vi "Scale Output ADXL345.vi"(9 "Byte1":u8, 11 "Byte0":u8) -> (3 "G's":fxp<+/-,32,10>)   [LabVIEW 2015]
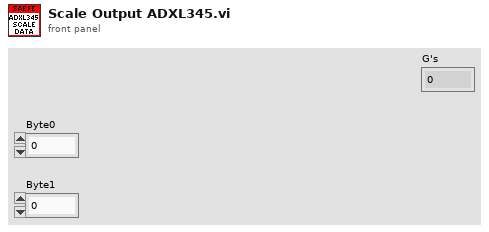
[diagram p1: front panel]
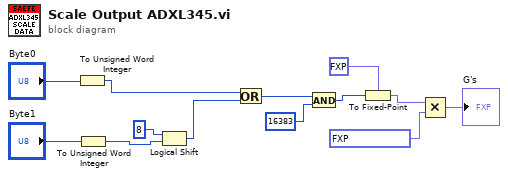
[diagram p0: block diagram]
diagram:
  n1 = To Unsigned Word Integer(number="Byte0") -> (unsigned 16bit integer=w9:u16)
  n2 = To Unsigned Word Integer(number="Byte1") -> (unsigned 16bit integer=w11:u16)
  n3 = Logical Shift(y=i16 8, x=w11) -> (x << y=w8:u16)
  n4 = Or(x=w9, y=w8) -> (x .or. y?=w7:u16)
  n5 = And(x=w7, y=u16 16383) -> (x .and. y?=w3:u16)
  n6 = To Fixed-Point(fixed-point type=fxp<+/-,16,16> 0.0, number=w3) -> (fixed-point=w1:fxp<+/-,16,16>)
  n7 = Multiply(x=w1, y=fxp<+,16,4> 3.89990234375) -> (x*y=→"G's":fxp<+/-,32,10>)
